vi "Articulate Control.vi"(8 "Second POV":i16, 9 "POV":i16, 10 "Left Articulate Target":dbl=0.5 format="%#_13g", 11 "Right Articulate Target":dbl=0.5 format="%#_13g") -> (1 "Left Art Output":dbl, 2 "Right Art Output":dbl)   [LabVIEW 2015]
panel:
  out "Right Rate":dbl
  out "Left Rate":dbl
  in  "Position Axis Right":dbl[](array[numeric])=[-1000.0, 0.0, 500.0, 1000.0]
  in  "Motor Effort Axis Right":dbl[](array[numeric])=[0.0, 0.0, 0.0, 0.0]
  in  "Position Axis Left":dbl[](array[numeric])=[-1000.0, 0.0, 500.0, 1000.0]
  in  "Motor Effort Axis Left":dbl[](array[numeric])=[0.0, 0.0, 0.0, 0.0]
  in  "Left Articulate OL":bool=TRUE
  in  "Left Art Control Inputs":T1={"Kp"=0.576, "Ki"=0.02875, "i upper"=0.0, "i lower"=0.0, "Output upper"=0.25, "Output lower"=-0.25}
  out "Left Articulate":cluster{"Articulate Target":dbl, "Feedback":dbl}
  in  "Right Articulate OL":bool=TRUE
  in  "Right Art Control Inputs":T1={"Kp"=0.576, "Ki"=0.02875, "i upper"=0.0, "i lower"=0.0, "Output upper"=0.25, "Output lower"=-0.25}
  out "Right Articulate":cluster{"Articulate Target":dbl, "Feedback":dbl}
  # "PI inputs and \nlimits"
  # "Feedforward inputs"
  # "Left Articulate Target"
  # "POV Value"
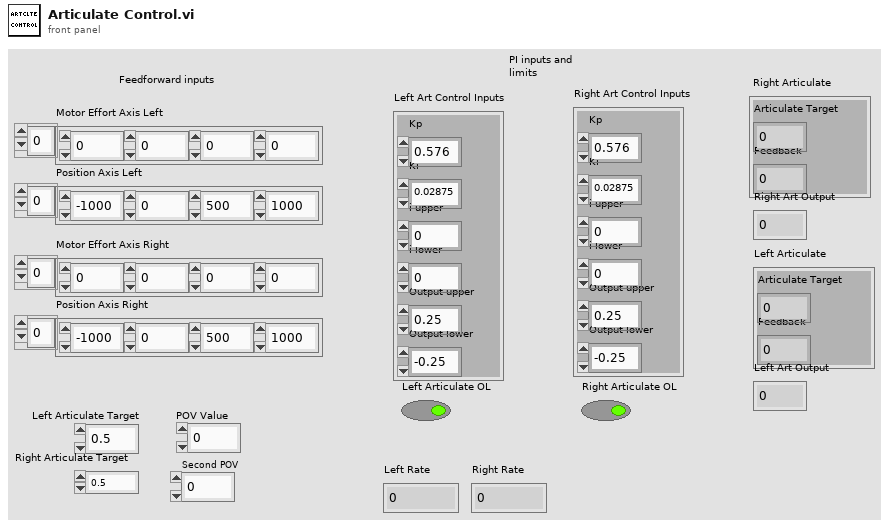
[diagram p1: front panel]
types:
  T1 = cluster{"Kp":dbl, "Ki":dbl, "i upper":dbl, "i lower":dbl, "Output upper":dbl, "Output lower":dbl}
  T2 = typedef "WPI_EncoderDevRef.ctl" = cluster{"DevStatus":errorcluster, "EncoderIndex":T3, "CounterIndex":T4, "DistancePerCount":dbl, "Decoding Type":T5}
  T3 = typedef "FPGA_EncoderIdx.ctl" = enum8{"Enc 0", "Enc 1", "Enc 2", "Enc 3", "Enc 4", "Enc 5", "Enc 6", "Enc 7", "Invalid"}
  T4 = typedef "FPGA_CounterCtrSystemIndex.ctl" = enum8{"Ctr 0", "Ctr 1", "Ctr 2", "Ctr 3", "Ctr 4", "Ctr 5", "Ctr 6", "Ctr 7", "Invalid"}
  T5 = typedef "WPI_EncoderType.ctl" = enum16{"1x", "2x", "4x"}
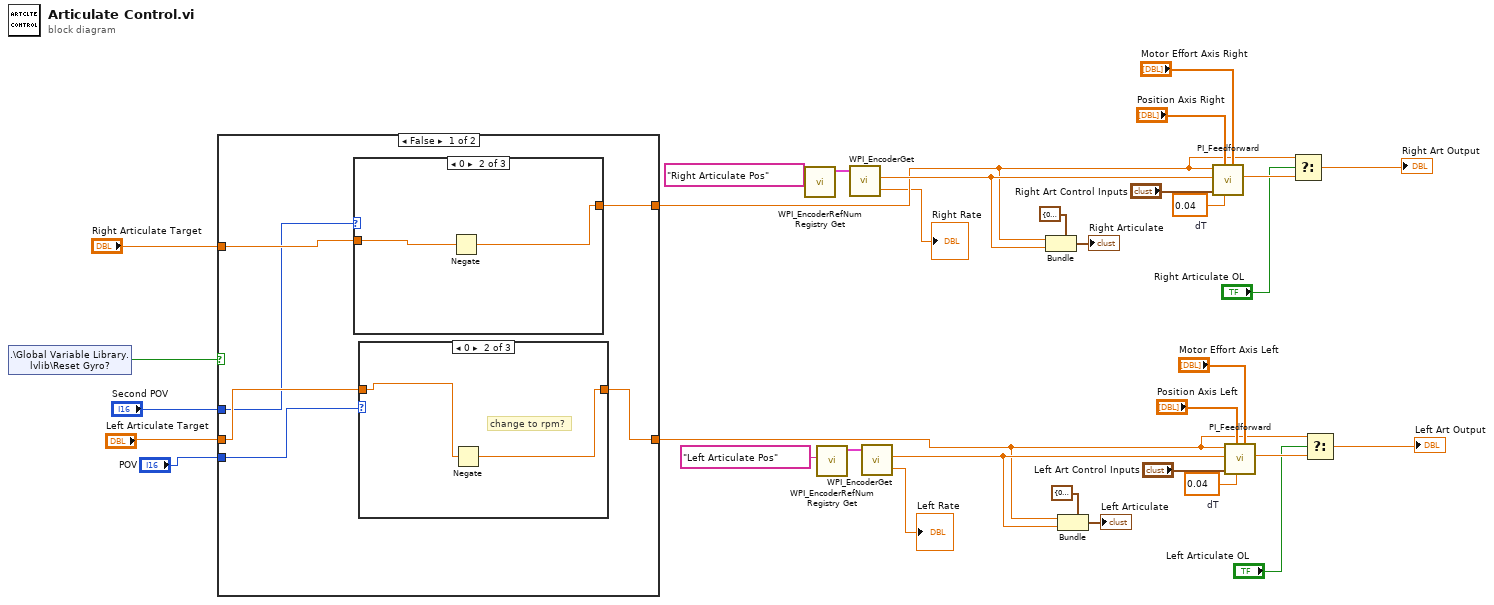
[diagram p0: block diagram]
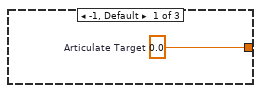
[diagram p2: hidden frame]
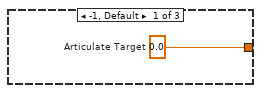
[diagram p4: hidden frame]
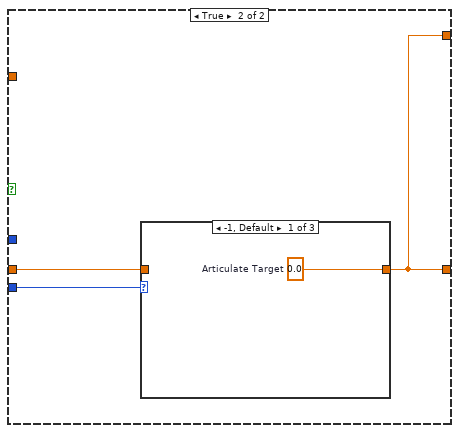
[diagram p6: hidden frame]
diagram:
  w13 = 0.04  # dT
  w25 = 0.04  # dT
  n1 = shared-variable ".\\Global Variable Library.lvlib\\Reset Gyro?"() -> (w33:bool)  [unwired: 1 in, 1 out]
  n2 = case shown="False" w33 {
    tunnel: [w39 w50] -> w8
    tunnel: [w38 w50] -> w7
    tunnel: "Left Articulate Target" -> [w37 w49]
    tunnel: "Right Articulate Target" -> [w36 _]
    tunnel: "POV" -> [w35 w48]
    tunnel: "Second POV" -> [w34 _]
    frame False {
      n3 = case shown="0" w34 {
        tunnel: [w40 w41 w43] -> w38
        tunnel: w36 -> [_ w42 w43]
        frame -1, Default {
          w40 = 0.0  # Articulate Target
        }
        frame 0 {
          n4 = Negate(x=w42) -> (-x=w41:dbl)
        }
        frame 180 {
        }
      }
      n5 = case shown="0" w35 {
        tunnel: [w44 w45 w47] -> w39
        tunnel: w37 -> [_ w46 w47]
        frame -1, Default {
          w44 = 0.0  # Articulate Target
        }
        frame 0 {
          # "change to rpm?"
          n6 = Negate(x=w46) -> (-x=w45:dbl)
        }
        frame 180 {
        }
      }
    }
    frame True {
      n7 = case shown="-1, Default" w48 {
        tunnel: [w51 w52 w53] -> w50
        tunnel: w49 -> [_ w52 w53]
        frame -1, Default {
          w51 = 0.0  # Articulate Target
        }
        frame 0 {
          # "change to rpm?"
        }
        frame 180 {
        }
      }
    }
  }
  n8 = call <vilib>:"WPI_EncoderRefNum Registry Get.vi"("refnum name"="Right Articulate Pos") -> ("EncoderDevRef"=w30:T2)  [unwired: 9 in, 1 out]
  n9 = call <vilib>:"WPI_EncoderRefNum Registry Get.vi"("refnum name"="Left Articulate Pos") -> ("EncoderDevRef"=w18:T2)  [unwired: 9 in, 1 out]
  n10 = call <vilib>:"WPI_EncoderGet.vi"("EncoderDevRef"=w30) -> ("Distance"=w28:dbl, "Rate"=→"Right Rate":dbl)  [unwired: 5 in, 4 out]
  n11 = call <vilib>:"WPI_EncoderGet.vi"("EncoderDevRef"=w18) -> ("Distance"=w16:dbl, "Rate"=→"Left Rate":dbl)  [unwired: 5 in, 4 out]
  n12 = Bundle(cluster=cluster{"Articulate Target":dbl, "Distance":dbl} {"Articulate Target"=0.0, "Distance"=0.0}, "Articulate Target"=w7, "Distance"=w28) -> (→"Right Articulate":cluster{"Articulate Target":dbl, "Distance":dbl})
  n13 = Bundle(cluster=cluster{"Articulate Target":dbl, "Distance":dbl} {"Articulate Target"=0.0, "Distance"=0.0}, "Articulate Target"=w8, "Distance"=w16) -> (→"Left Articulate":cluster{"Articulate Target":dbl, "Distance":dbl})
  n14 = call "PI_Feedforward.vi"("Motor Effort Axis"="Motor Effort Axis Right", "dT"=w25, "Position Axis"="Position Axis Right", "Control Inputs"="Right Art Control Inputs", "Feed Back"=w28, "Target"=w7) -> ("Output"=w23:dbl)  [unwired: 3 in, 2 out]
  n15 = call "PI_Feedforward.vi"("Motor Effort Axis"="Motor Effort Axis Left", "dT"=w13, "Position Axis"="Position Axis Left", "Control Inputs"="Left Art Control Inputs", "Feed Back"=w16, "Target"=w8) -> ("Output"=w11:dbl)  [unwired: 3 in, 2 out]
  n16 = Select(t=w7, s="Right Articulate OL", f=w23) -> (s? t:f=→"Right Art Output":dbl)
  n17 = Select(t=w8, s="Left Articulate OL", f=w11) -> (s? t:f=→"Left Art Output":dbl)
